vi "虚拟放射源设置.vi"(1 "信号输出":bool, 2 "放大倍数":dbl min=0.0 max=2.0, 4 "错误输入（无错误）":errorcluster, 5 "最小时间间隔":u16=20 min=15 step=1, 6 "计数率":u32=20 max=2000000, 7 "VISA资源名称":refnum<visa-resource-name>) -> (0 "错误输出":errorcluster, 3 "VISA资源名称输出":refnum<visa-resource-name>)   [LabVIEW 2014]
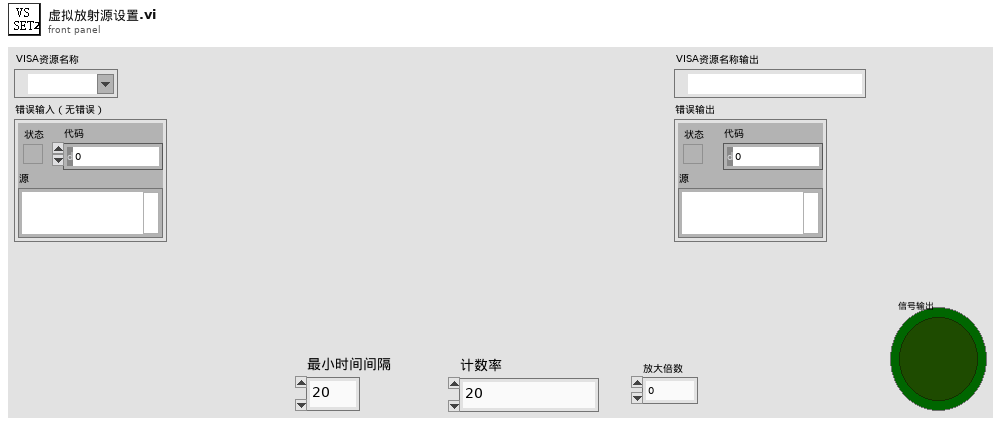
[diagram p1: front panel]
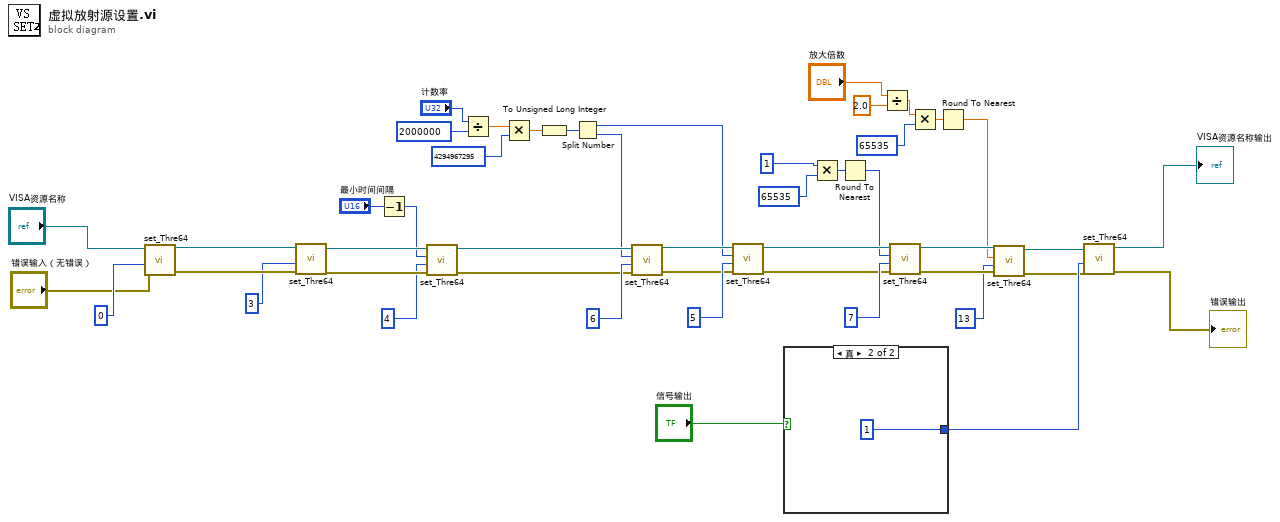
[diagram p0: block diagram]
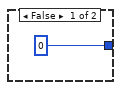
[diagram p2: hidden frame]
diagram:
  n1 = call "set_Thre64.vi"("错误输入（无错误）"="错误输入（无错误）", "命令"=0, "VISA资源名称"="VISA资源名称") -> ("错误输出"=w46:errorcluster, "VISA资源名称输出"=w47:refnum<visa-resource-name>)  [unwired: 7 in]
  n2 = call "set_Thre64.vi"("错误输入（无错误）"=w46, "命令"=3, "VISA资源名称"=w47) -> ("错误输出"=w44:errorcluster, "VISA资源名称输出"=w45:refnum<visa-resource-name>)  [unwired: 7 in]
  n3 = Decrement(x="最小时间间隔") -> (x-1=w40:u16)
  n4 = call "set_Thre64.vi"("错误输入（无错误）"=w44, "命令"=4, "数字"=w40, "VISA资源名称"=w45) -> ("错误输出"=w38:errorcluster, "VISA资源名称输出"=w39:refnum<visa-resource-name>)  [unwired: 6 in]
  n5 = Divide(x="计数率", y=u32 2000000) -> (x/y=w35:dbl)
  n6 = Multiply(x=w35, y=u32 4294967295) -> (x*y=w30:dbl)
  n7 = To Unsigned Long Integer(number=w30) -> (unsigned 32bit integer=w29:u32)
  n8 = Split Number(x=w29) -> (hi(x)=w27:u16, lo(x)=w28:u16)
  n9 = call "set_Thre64.vi"("错误输入（无错误）"=w38, "命令"=6, "数字"=w28, "VISA资源名称"=w39) -> ("错误输出"=w31:errorcluster, "VISA资源名称输出"=w32:refnum<visa-resource-name>)  [unwired: 6 in]
  n10 = call "set_Thre64.vi"("错误输入（无错误）"=w31, "命令"=5, "数字"=w27, "VISA资源名称"=w32) -> ("错误输出"=w24:errorcluster, "VISA资源名称输出"=w25:refnum<visa-resource-name>)  [unwired: 6 in]
  n11 = case shown="真" "信号输出" {
    tunnel: [0 1] -> w16
    frame False {
    }
    frame True {
    }
  }
  n12 = Multiply(x=1, y=u32 65535) -> (x*y=w22:u32)
  n13 = Round To Nearest(number=w22) -> (nearest integer value=w21:u32)
  n14 = Divide(x="放大倍数", y=2.0) -> (x/y=w5:dbl)
  n15 = call "set_Thre64.vi"("错误输入（无错误）"=w24, "命令"=7, "数字"=w21, "VISA资源名称"=w25) -> ("错误输出"=w11:errorcluster, "VISA资源名称输出"=w13:refnum<visa-resource-name>)  [unwired: 6 in]
  n16 = Multiply(x=w5, y=u32 65535) -> (x*y=w7:dbl)
  n17 = Round To Nearest(number=w7) -> (nearest integer value=w3:dbl)
  n18 = call "set_Thre64.vi"("错误输入（无错误）"=w11, "命令"=u8 13, "数字"=w3, "VISA资源名称"=w13) -> ("错误输出"=w10:errorcluster, "VISA资源名称输出"=w12:refnum<visa-resource-name>)  [unwired: 6 in]
  n19 = call "set_Thre64.vi"("错误输入（无错误）"=w10, "命令"=w16, "VISA资源名称"=w12) -> ("错误输出"=→"错误输出":errorcluster, "VISA资源名称输出"=→"VISA资源名称输出":refnum<visa-resource-name>)  [unwired: 7 in]
